vi "BlockFrequencyTooHigh.vi"(8 "error in (no error)":errorcluster) -> (0 "error out":errorcluster, 3 "BFTH":bool)   [LabVIEW 2015, in "ESLSCDLL.lvlib"]
uses:
  ESLSCDLL.lvlib
  Globals.vi
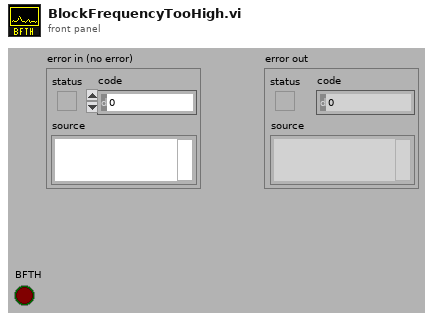
[diagram p1: front panel]
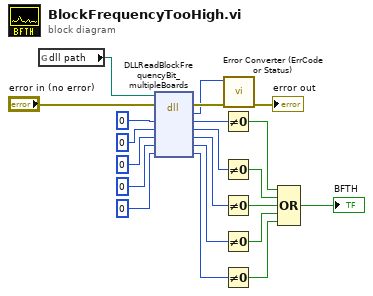
[diagram p0: block diagram]
diagram:
  n1 = global read "Globals.vi" "dll path"() -> (w1:path)
  n2 = dll-call lib="C:/ENTW/PCIE/LV64/board.vis/ESLSCDLL.dll" fn="DLLReadBlockFrequencyBit_multipleBoards" ("lwlscdll.dll:DLLWriteLongS0")(path in=w1, error in="error in (no error)", "blockFrequencyTooHigh0"=u8 0 ("scanFrequencyTooHigh"), "blockFrequencyTooHigh1"=u8 0, "blockFrequencyTooHigh2"=u8 0, "blockFrequencyTooHigh3"=u8 0, "blockFrequencyTooHigh4"=u8 0) -> (error out=w19:errorcluster, "es_status_codes"=w18:i32, "blockFrequencyTooHigh0"=w17:u8, "blockFrequencyTooHigh1"=w11:u8, "blockFrequencyTooHigh2"=w10:u8, "blockFrequencyTooHigh3"=w9:u8, "blockFrequencyTooHigh4"=w8:u8)  [unwired: 1 in, 1 out]
  n3 = Not Equal To 0?(x=w17) -> (x != 0?=w7:bool)
  n4 = Not Equal To 0?(x=w11) -> (x != 0?=w6:bool)
  n5 = Not Equal To 0?(x=w10) -> (x != 0?=w5:bool)
  n6 = Not Equal To 0?(x=w9) -> (x != 0?=w4:bool)
  n7 = Not Equal To 0?(x=w8) -> (x != 0?=w3:bool)
  n8 = call "Error Converter (ErrCode or Status).vi"("error in (no error)"=w19, "error code"=w18) -> ("error out"=→"error out":errorcluster)  [unwired: 9 in]
  n9 = Compound Arithmetic op=OR(w7, w6, w5, w4, w3) -> (→"BFTH":bool)
